vi "LoopTable.vi"() -> ()   [LabVIEW 2015]
panel:
  in  "Loop table":string[][](table)
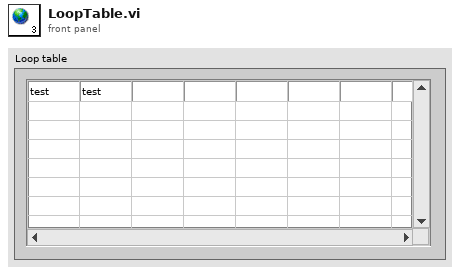
[diagram p1: front panel]
diagram:
